vi "TestExec.Parse Barcode to PN and SN.vi"(9 "Barcode PN SN Format":T1={"Type"=enum."SN_Only", "Len"=12, "Delimiter"="TAB"}, 11 "Barcode":string) -> (1 "PN":string, 3 "SN":string)   [LabVIEW 2018]
uses:
  Controls and Type Defs/TestExec.Barcode PN SN Format Type.ctl
panel:
  out "Delim":string="TAB"
  # "TAB CR LF EOL(CRLF)"
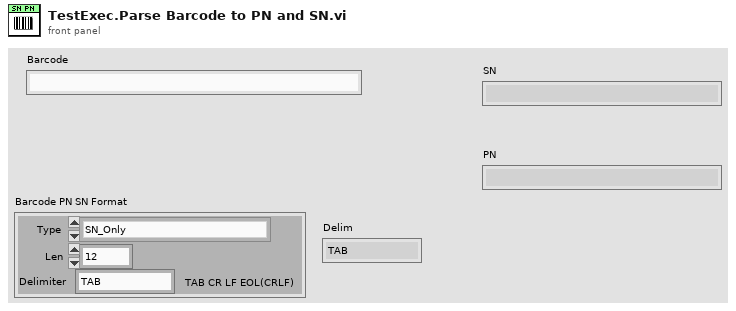
[diagram p1: front panel]
types:
  T1 = typedef "TestExec.Barcode PN SN Format Type.ctl" = cluster{"Type":enum16{"SN_Only", "SN_PN_LenDelim", "PN_SN_LenDelim", "SN_PN_StrDelim", "PN_SN_StrDelim"}, "Len":i32, "Delimiter":string}
  T2 = enum16{"SN_Only", "SN_PN_LenDelim", "PN_SN_LenDelim", "SN_PN_StrDelim", "PN_SN_StrDelim"}
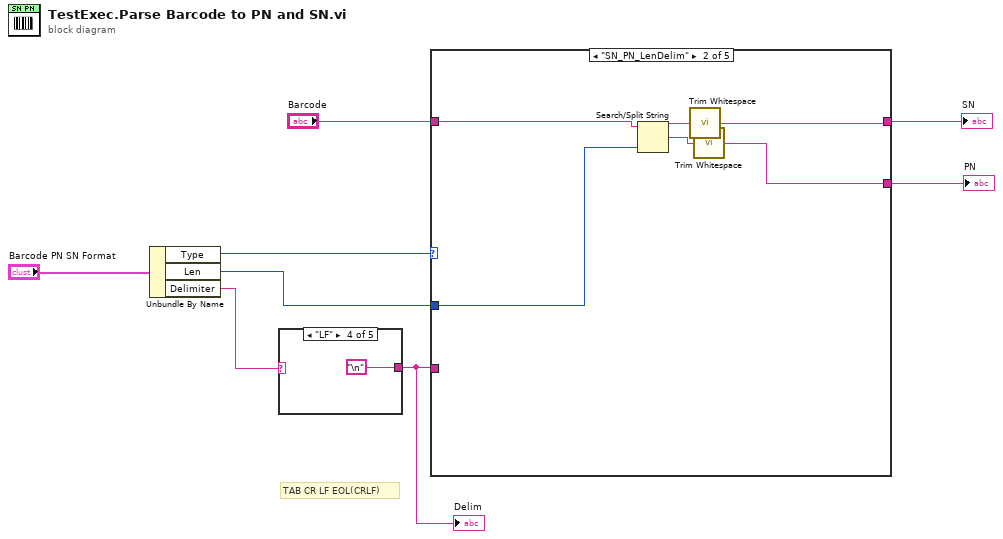
[diagram p0: block diagram]
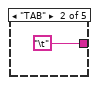
[diagram p3: hidden frame]
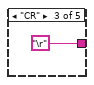
[diagram p4: hidden frame]
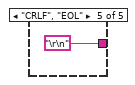
[diagram p5: hidden frame]
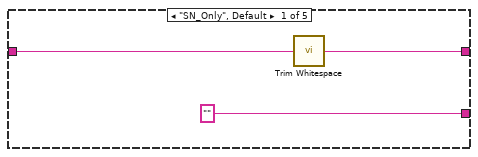
[diagram p6: hidden frame]
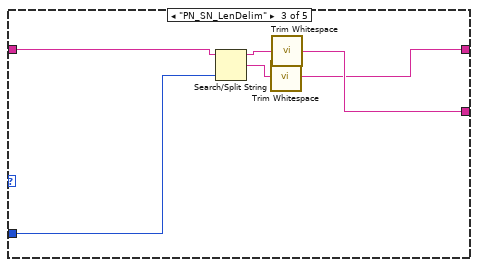
[diagram p7: hidden frame]
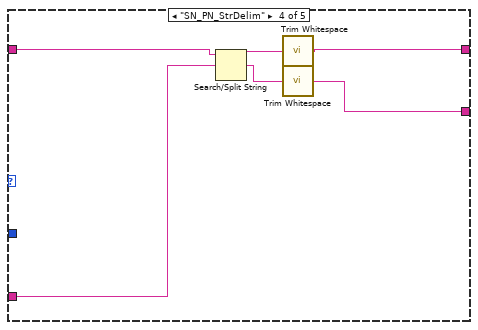
[diagram p8: hidden frame]
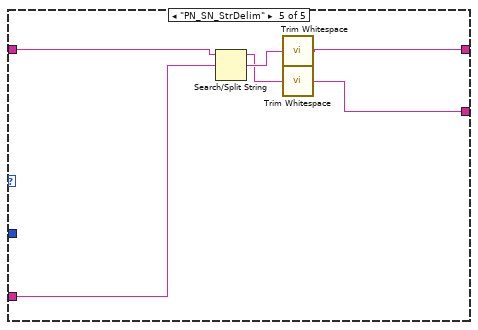
[diagram p9: hidden frame]
diagram:
  # "TAB CR LF EOL(CRLF)"
  n1 = Unbundle By Name("Barcode PN SN Format") -> ("Type"=w3:T2, "Len"=w2:i32, "Delimiter"=w1:string)
  n2 = case shown="\"LF\"" w1 {
    selector: w1 -> [w9 _ _ _ _]
    tunnel: [w9 "\t" "\r" "\n" "\r\n"] -> w5
    frame Default {
    }
    frame "TAB" {
    }
    frame "CR" {
    }
    frame "LF" {
    }
    frame "CRLF", "EOL" {
    }
  }
  "Delim" <- w5
  n3 = case shown="\"SN_PN_LenDelim\"" w3 {
    tunnel: w2 -> [_ w21 w27 _ _]
    tunnel: w5 -> [_ _ _ w33 w39]
    tunnel: "Barcode" -> [w16 w22 w28 w34 w40]
    tunnel: [w15 w19 w23 w29 w37] -> w7
    tunnel: ["" w17 w24 w30 w38] -> w6
    frame "SN_Only", Default {
      n4 = call <vilib>:"Trim Whitespace.vi"("string"=w16) -> ("trimmed string"=w15:string)  [unwired: 1 in]
    }
    frame "SN_PN_LenDelim" {
      n5 = Search/Split String(string=w22, offset (0)=w21) -> (substring before match=w20:string, match + rest of string=w18:string)  [unwired: 1 in, 1 out]
      n6 = call <vilib>:"Trim Whitespace.vi"("string"=w20) -> ("trimmed string"=w19:string)  [unwired: 1 in]
      n7 = call <vilib>:"Trim Whitespace.vi"("string"=w18) -> ("trimmed string"=w17:string)  [unwired: 1 in]
    }
    frame "PN_SN_LenDelim" {
      n8 = Search/Split String(string=w28, offset (0)=w27) -> (substring before match=w26:string, match + rest of string=w25:string)  [unwired: 1 in, 1 out]
      n9 = call <vilib>:"Trim Whitespace.vi"("string"=w25) -> ("trimmed string"=w23:string)  [unwired: 1 in]
      n10 = call <vilib>:"Trim Whitespace.vi"("string"=w26) -> ("trimmed string"=w24:string)  [unwired: 1 in]
    }
    frame "SN_PN_StrDelim" {
      n11 = Search/Split String(string=w34, search string/char (-)=w33) -> (substring before match=w32:string, match + rest of string=w31:string)  [unwired: 1 in, 1 out]
      n12 = call <vilib>:"Trim Whitespace.vi"("string"=w32) -> ("trimmed string"=w29:string)  [unwired: 1 in]
      n13 = call <vilib>:"Trim Whitespace.vi"("string"=w31) -> ("trimmed string"=w30:string)  [unwired: 1 in]
    }
    frame "PN_SN_StrDelim" {
      n14 = Search/Split String(string=w40, search string/char (-)=w39) -> (substring before match=w35:string, match + rest of string=w36:string)  [unwired: 1 in, 1 out]
      n15 = call <vilib>:"Trim Whitespace.vi"("string"=w36) -> ("trimmed string"=w37:string)  [unwired: 1 in]
      n16 = call <vilib>:"Trim Whitespace.vi"("string"=w35) -> ("trimmed string"=w38:string)  [unwired: 1 in]
    }
  }
  "SN" <- w7
  "PN" <- w6
